vi "(Depricated) Close.vi"(6 "Interlock Chain":refnum<class "Interlock.lvclass">[](array[class]), 8 "error in (no error)":errorcluster, 10 "Index (All -1)":i32=-1, 11 "Valve in":refnum<class "Valve.lvclass">=refnum) -> (0 "error out":errorcluster, 3 "Valve out":refnum<class "Valve.lvclass">)   [LabVIEW 2015]
uses:
  Valve.lvclass
  Interlocks/Interlock/Interlock.lvclass
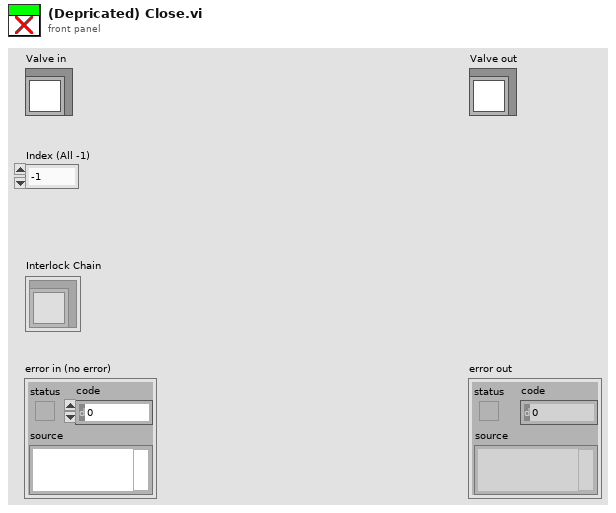
[diagram p1: front panel]
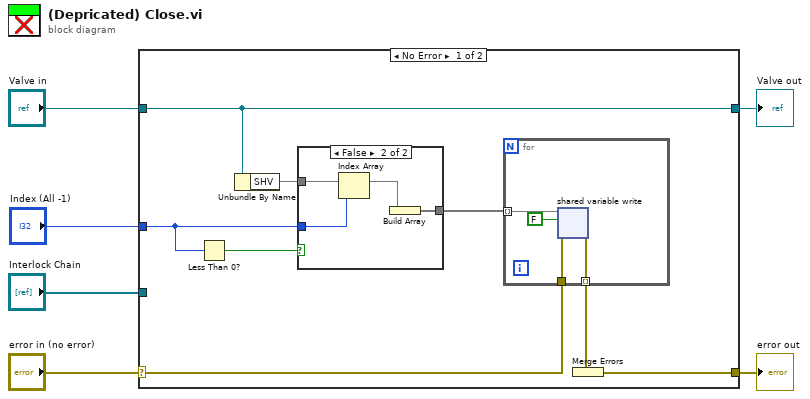
[diagram p0: block diagram]
diagram:
  n1 = case shown="No Error" "error in (no error)" {
    selector: "error in (no error)" -> [w13 w25]
    tunnel: [w7 w25] -> w5
    tunnel: [w14 w24] -> w3
    tunnel: "Valve in" -> [w14 w24]
    tunnel: "Interlock Chain" -> [_ _]
    tunnel: "Index (All -1)" -> [w8 _]
    frame No Error {
      n2 = Less Than 0?(x=w8) -> (x < 0?=w9:bool)
      n3 = Unbundle By Name(w14) -> ("SHV"=w11)
      n4 = case shown="False" w9 {
        tunnel: w11 -> [w15 w19]
        tunnel: [w15 w18] -> w10
        tunnel: w8 -> [_ w17]
        frame True {
        }
        frame False {
          n5 = Index Array(array=w19, index=w17) -> (element=w16)
          n6 = Build Array(w16) -> (w18:void[])
        }
      }
      n7 = for {
        tunnel: w13 -> [w22]
        tunnel: [w21] -> w12 mode=indexing
        tunnel: w10 -> [w20] mode=indexing
        n8 = shared-variable-write(w20, w22, FALSE) -> (w21:errorcluster)  [unwired: 1 out]
      }
      n9 = Merge Errors(w12) -> (w7:errorcluster)
    }
    frame Error {
    }
  }
  "error out" <- w5
  "Valve out" <- w3
